vi "test - Sync param Value to the top INI.vi"(8 "error in (no error)":errorcluster, 11 "TestCase in":refnum<class "csm-ini-variable-addon.lvclass">) -> (0 "error out":errorcluster, 3 "TestCase out":refnum<class "csm-ini-variable-addon.lvclass">)   [LabVIEW 2017, in "csm-ini-variable-addon.lvclass"]
uses:
  csm-ini-variable-addon.lvclass
  9da69169-e459-4de5-bd52-65d5bd10cfe3.vi
  819d10de-cc93-4901-8476-a53ff0da62fe.vi
  4331c652-d221-4445-b443-08c445718bf9.vi
  9da69169-e459-4de5-bd52-65d5bd10cfe3.vi/99de0c97-112a-4c86-9094-c187659127e1.vi
  <vilib>/Utility/error.llb/Clear Errors.vi
  819d10de-cc93-4901-8476-a53ff0da62fe.vi/b09b9099-6be0-413b-8afc-4908471460c3.vi
  INI-Static-Variable-Support/_Support/FlagInstance-CSMINIVariable.vi
  4331c652-d221-4445-b443-08c445718bf9.vi/b09b9099-6be0-413b-8afc-4908471460c3.vi
  <userlib>/_NEVSTOP/Communicable State Machine(CSM)/_Support/ChangeFlag/ChangeFlag-Read.vi
  <vilib>/Utility/Data Type/Get Type Information.vi
  <userlib>/_NEVSTOP/Communicable State Machine(CSM)/addons/API-String-Arugments-Support/_Support/Data To SingleElementsArray_csm.vi
  <userlib>/_NEVSTOP/Communicable State Machine(CSM)/addons/API-String-Arugments-Support/_Support/Data To API String Arguments.vi
  INI-Static-Variable-Support/_Support/Parse Used Session and Name.vi
  INI-Static-Variable-Support/_Support/INI-FGV(lvlibp).vi
  <userlib>/_NEVSTOP/Communicable State Machine(CSM)/_Support/ChangeFlag/ChangeFlagDB.vi
  INI-Static-Variable-Support/_Support/Populate String with INI Variable.vi
  <userlib>/_NEVSTOP/Communicable State Machine(CSM)/addons/API-String-Arugments-Support/_Support/Convert API String Arguments to Data(variant).vi
  <userlib>/_NEVSTOP/Communicable State Machine(CSM)/addons/API-String-Arugments-Support/_Support/SingleElementsArray To Data_csm.vi
  INI-Static-Variable-Support/INI-Static-Variable-Support.lvlib
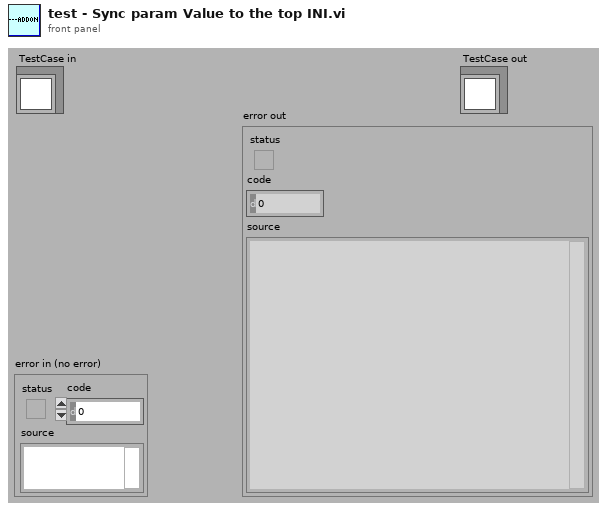
[diagram p1: front panel]
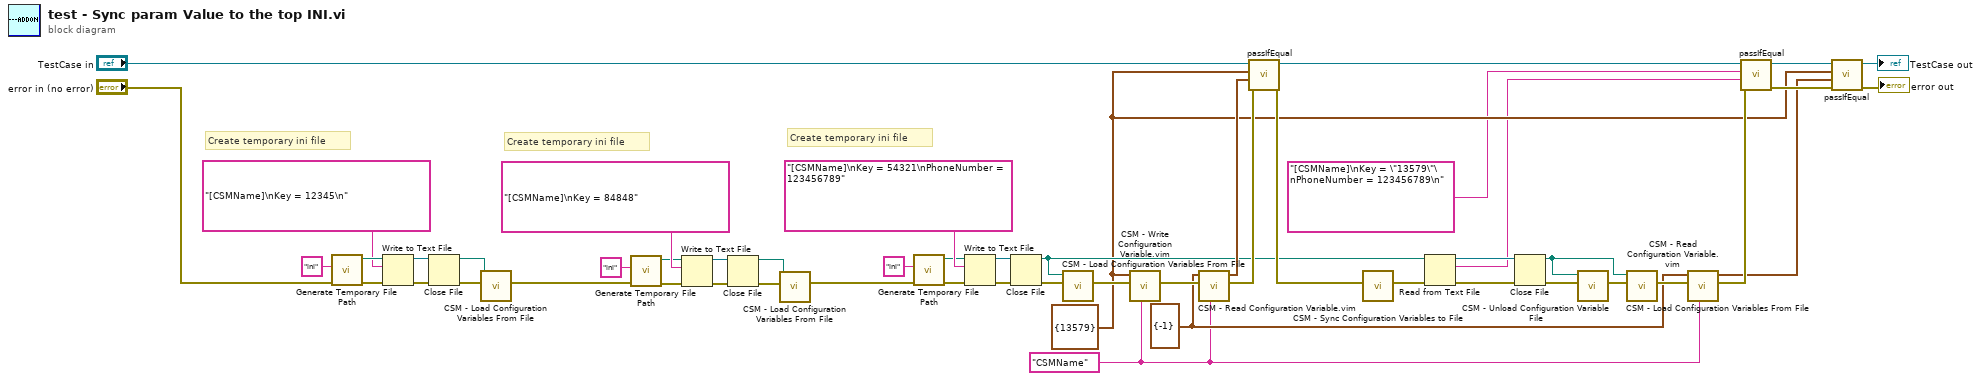
[diagram p0: block diagram]
diagram:
  w11 = cluster{"Key":i32} {"Key"=-1}
  w4 = cluster{"Key":i32} {"Key"=13579}
  w10 = "CSMName" ("Section Name(\"\" as Default)")
  # "Create temporary ini file"
  # "Create temporary ini file"
  # "Create temporary ini file"
  n1 = call <vilib>:"Generate Temporary File Path.vi"("error in (no error)"="error in (no error)", "Temporary File Extension (tmp)"="ini") -> ("error out"=w51:errorcluster, "Unique Temporary File Path"=w48:path)  [unwired: 8 in]
  n2 = Write to Text File(file (use dialog)=w48, text="[CSMName]\nKey = 12345\n", error in=w51) -> (refnum out=w47:refnum<file>, error out=w49:errorcluster)  [unwired: 1 in, 1 out]
  n3 = Close File(refnum=w47, error in=w49) -> (path=w28:path, error out=w46:errorcluster)
  n4 = call "CSM - Load Configuration Variables From File.vi"("error in (no error)"=w46, "Configuration Path"=w28) -> ("error out"=w17:errorcluster)  [unwired: 7 in]
  n5 = call <vilib>:"Generate Temporary File Path.vi"("error in (no error)"=w17, "Temporary File Extension (tmp)"="ini") -> ("error out"=w18:errorcluster, "Unique Temporary File Path"=w21:path)  [unwired: 8 in]
  n6 = Write to Text File(file (use dialog)=w21, text="[CSMName]\nKey = 84848", error in=w18) -> (refnum out=w22:refnum<file>, error out=w20:errorcluster)  [unwired: 1 in, 1 out]
  n7 = Close File(refnum=w22, error in=w20) -> (path=w25:path, error out=w23:errorcluster)
  n8 = call "CSM - Load Configuration Variables From File.vi"("error in (no error)"=w23, "Configuration Path"=w25) -> ("error out"=w16:errorcluster)  [unwired: 7 in]
  n9 = call <vilib>:"Generate Temporary File Path.vi"("error in (no error)"=w16, "Temporary File Extension (tmp)"="ini") -> ("error out"=w38:errorcluster, "Unique Temporary File Path"=w41:path)  [unwired: 8 in]
  n10 = Write to Text File(file (use dialog)=w41, text="[CSMName]\nKey = 54321\nPhoneNumber = 123456789", error in=w38) -> (refnum out=w42:refnum<file>, error out=w40:errorcluster)  [unwired: 1 in, 1 out]
  n11 = Close File(refnum=w42, error in=w40) -> (path=w29:path, error out=w43:errorcluster)
  n12 = call "CSM - Load Configuration Variables From File.vi"("error in (no error)"=w43, "Configuration Path"=w29) -> ("error out"=w37:errorcluster)  [unwired: 7 in]
  n13 = call "CSM - Write Configuration Variable.vim"("Section Name (\"\" as Default)"=w10, "error in (no error)"=w37, "Configuration"=w4) -> ("error out"=w35:errorcluster)  [unwired: 5 in, 1 out]
  n14 = call "CSM - Read Configuration Variable.vim"("Section Name (\"\" as Default)"=w10, "error in (no error)"=w35, "Configuration Prototype (Cluster Prefered)"=w11) -> ("error out"=w31:errorcluster, "Configuration"=w32:cluster{"Key":i32})  [unwired: 5 in]
  n15 = call-dynamic "passIfEqual.vi"("error in (no error)"=w31, "y"=w32, "x"=w4, "TestCase in"="TestCase in") -> ("error out"=w30:errorcluster, "TestCase out"=w33:refnum<class "csm-ini-variable-addon.lvclass">)  [unwired: 6 in]
  n16 = call "CSM - Sync Configuration Variables to File.vi"("error in (no error)"=w30) -> ("error out"=w36:errorcluster)  [unwired: 8 in]
  n17 = Read from Text File(file (use dialog)=w29, error in=w36) -> (refnum out=w27:refnum<file>, text=w1:string, error out=w26:errorcluster)  [unwired: 2 in, 1 out]
  n18 = Close File(refnum=w27, error in=w26) -> (path=w13:path, error out=w15:errorcluster)
  n19 = call "CSM - Unload Configuration Variable File.vi"("error in (no error)"=w15, "Path"=w13) -> ("error out"=w14:errorcluster)  [unwired: 7 in]
  n20 = call "CSM - Load Configuration Variables From File.vi"("error in (no error)"=w14, "Configuration Path"=w13) -> ("error out"=w12:errorcluster)  [unwired: 7 in]
  n21 = call "CSM - Read Configuration Variable.vim"("Section Name (\"\" as Default)"=w10, "error in (no error)"=w12, "Configuration Prototype (Cluster Prefered)"=w11) -> ("error out"=w9:errorcluster, "Configuration"=w3:cluster{"Key":i32})  [unwired: 5 in]
  n22 = call-dynamic "passIfEqual.vi"("error in (no error)"=w9, "y"=w1, "x"="[CSMName]\nKey = \"13579\"\nPhoneNumber = 123456789\n", "TestCase in"=w33) -> ("error out"=w7:errorcluster, "TestCase out"=w8:refnum<class "csm-ini-variable-addon.lvclass">)  [unwired: 6 in]
  n23 = call-dynamic "passIfEqual.vi"("error in (no error)"=w7, "y"=w3, "x"=w4, "TestCase in"=w8) -> ("error out"=→"error out":errorcluster, "TestCase out"=→"TestCase out":refnum<class "csm-ini-variable-addon.lvclass">)  [unwired: 6 in]
